vi "Auto Kettle Final.vi"() -> ()   [LabVIEW 2023]
uses:
  <vilib>/MakerHub/LINX/Public/Peripherals/Digital/Digital Read 1 Chan.vi
  <vilib>/MakerHub/LINX/Public/Peripherals/Digital/Digital Write 1 Chan.vi
  <vilib>/MakerHub/LINX/Public/Peripherals/Digital/Digital Read N Chans.vi
  <vilib>/MakerHub/LINX/Public/Peripherals/Digital/Digital Write N Chans.vi
  <vilib>/MakerHub/LINX/Private/Local IO/LinxDigitalRead.vi
  <vilib>/MakerHub/LINX/Public/Utilities/Check Channel.vi
  <vilib>/MakerHub/LINX/Private/Local IO/LinxDigitalWrite.vi
  <vilib>/MakerHub/LINX/Public/Utilities/Open Serial.vi
  <vilib>/MakerHub/LINX/Private/Utilties/Generate Error.vi
  <vilib>/MakerHub/LINX/LMH-LINX.lvlib
panel:
  out "Kettle OFF":bool
  in  "True":string
  in  "False":string
  out "Live LED":bool
  out "Error Out":errorcluster
  in  "Serial Port":refnum<visa-resource-name>="N/A"
  out "Measured Temperature":dbl
  out "Waveform Chart":dbl(graph)
  in  "stop":bool
  in  "Desired Temp":i32=40
  out "Kettle On":bool
  out "Kettle Temp":dbl(slide) scale=0.0..100.0
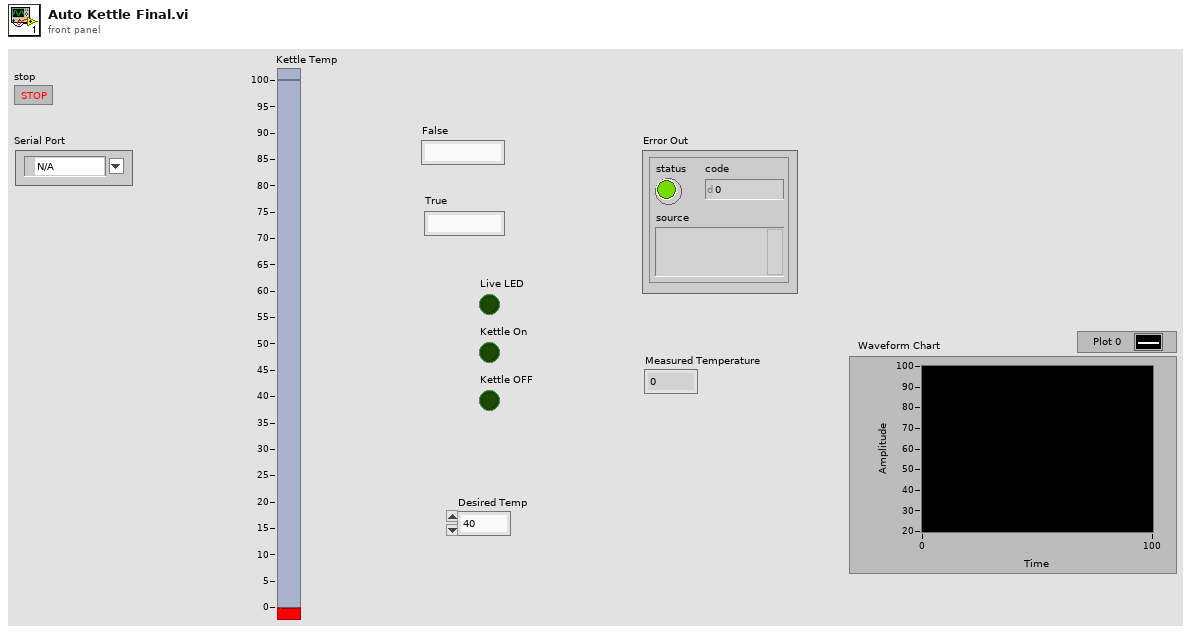
[diagram p1: front panel]
types:
  T1 = typedef "LMH-LINX.lvlib/LINX Ref.ctl" = cluster{"IO":T2, "Interface":T3, "LINX Device Config":T4}
  T2 = typedef "LMH-LINX.lvlib/Platform.ctl" = enum16{"Remote", "Local"}
  T3 = typedef "LMH-LINX.lvlib/Interface.ctl" = enum16{"Serial", "TCP"}
  T4 = typedef "LMH-LINX.lvlib/Device.lvlib/LINX Device Config.ctl" = cluster{"Interface":T3, "COM Port":refnum<visa-resource-name>, "TCP Configuration":T5, "Device Family":u8, "Device ID":u8, "Device Name":string, "TCP Ref":refnum<k5>, "Channels":T6}
  T5 = typedef "LMH-LINX.lvlib/Device.lvlib/TCP Config.ctl" = cluster{"IP Address":string, "Port":u16}
  T6 = typedef "LMH-LINX.lvlib/Channels.ctl" = cluster{"DI":u8[], "DO":u8[], "AI":u8[], "AO":u8[], "PWM":u8[], "QE":u8[], "UART":u8[], "I2C 2":u8[], "SPI":u8[], "CAN":u8[], "Servo":u8[], "AI Ref (V)":dbl, "AI Resolution (Bits)":u8, "AO Ref (V)":dbl, "AO Resolution (Bits)":u8}
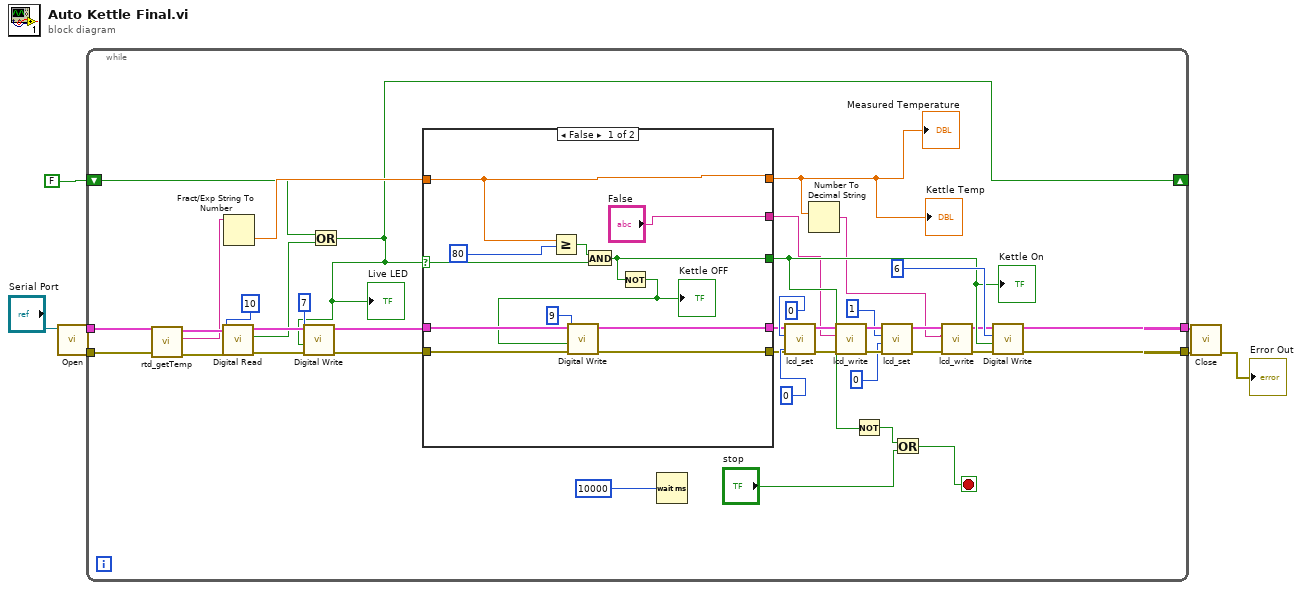
[diagram p0: block diagram]
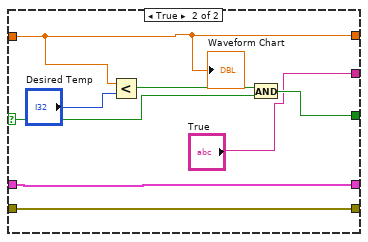
[diagram p2: hidden frame]
diagram:
  n1 = call-poly <vilib>:"Open.vi"("Serial Port"="Serial Port") -> ("Error Out"=w4:errorcluster, "LINX Resource"=w5:T1)  [unwired: 8 in, 1 out]
  n2 = while {
    shift-right: [w9] -> _
    shift-left: FALSE -> [w34]
    tunnel: w5 -> [w40]
    tunnel: w4 -> [w39]
    tunnel: [w20] -> w1
    tunnel: [w21] -> w2
    stop <- w45 stop-if-true
    n3 = call "rtd_getTemp.vi"("Error In"=w39, "LINX Resource"=w40) -> ("Error Out"=w38:errorcluster, "string"=w35:string, "LINX Resource 2"=w37:T1)  [unwired: 7 in]
    n4 = call-poly <vilib>:"Digital Read.vi"("Error In"=w38, "DI Channel"=10, "LINX Resource"=w37) -> ("Error Out"=w33:errorcluster, "DI Value"=w31:bool, "LINX Resource"=w32:T1)  [unwired: 6 in]
    n5 = Fract/Exp String To Number(string=w35) -> (number=w36:dbl)  [unwired: 3 in, 1 out]
    n6 = Or(x=w34, y=w31) -> (x .or. y?=w9:bool)
    "Live LED" <- w9
    n7 = call-poly <vilib>:"Digital Write.vi"("Error In"=w33, "Output Value"=w9, "DO Channel"=u8 7, "LINX Resource"=w32) -> ("Error Out"=w24:errorcluster, "LINX Resource"=w25:T1)  [unwired: 6 in]
    n8 = case shown="False" w9 {
      selector: w9 -> [w51 w62]
      tunnel: w36 -> [w57 w61]
      tunnel: [w57 w61] -> w8
      tunnel: [w49 w65] -> w41
      tunnel: w25 -> [w53 w63]
      tunnel: [w55 w63] -> w23
      tunnel: w24 -> [w52 w64]
      tunnel: [w54 w64] -> w22
      tunnel: ["False" "True"] -> w13
      frame False {
        n9 = Greater Or Equal?(x=w57, y=80 ("Numeric")) -> (x >= y?=w58:bool)
        n10 = And(x=w58, y=w51) -> (x .and. y?=w49:bool)
        n11 = Not(x=w49) -> (.not. x?=w48:bool)
        "Kettle OFF" <- w48
        n12 = call-poly <vilib>:"Digital Write.vi"("Error In"=w52, "Output Value"=w48, "DO Channel"=u8 9, "LINX Resource"=w53) -> ("Error Out"=w54:errorcluster, "LINX Resource"=w55:T1)  [unwired: 6 in]
      }
      frame True {
        n13 = Less?(x=w61, y="Desired Temp") -> (x < y?=w66:bool)
        n14 = And(x=w66, y=w62) -> (x .and. y?=w65:bool)
        "Waveform Chart" <- w61
      }
    }
    "Kettle Temp" <- w8
    "Kettle On" <- w41
    "Measured Temperature" <- w8
    n15 = Wait (ms)(milliseconds to wait=10000) -> ()  [unwired: 1 out]
    n16 = call "lcd_set.vi"("Error In"=w22, "Column"=0, "Row"=0, "LINX Resource"=w23) -> ("Error Out"=w27:errorcluster, "LINX Resource out"=w26:T1)  [unwired: 6 in]
    n17 = Number To Decimal String(number=w8) -> (decimal integer string=w12:string)  [unwired: 1 in]
    n18 = call "lcd_write.vi"("Error In"=w27, "string"=w13, "LINX Resource"=w26) -> ("Error Out"=w18:errorcluster, "LINX Resource out"=w19:T1)  [unwired: 7 in]
    n19 = Not(x=w41) -> (.not. x?=w46:bool)
    n20 = call "lcd_set.vi"("Error In"=w18, "Column"=0, "Row"=1, "LINX Resource"=w19) -> ("Error Out"=w17:errorcluster, "LINX Resource out"=w16:T1)  [unwired: 6 in]
    n21 = Or(x=w46, y="stop") -> (x .or. y?=w45:bool)
    n22 = call "lcd_write.vi"("Error In"=w17, "string"=w12, "LINX Resource"=w16) -> ("Error Out"=w15:errorcluster, "LINX Resource out"=w14:T1)  [unwired: 7 in]
    n23 = call-poly <vilib>:"Digital Write.vi"("Error In"=w15, "Output Value"=w41, "DO Channel"=6, "LINX Resource"=w14) -> ("Error Out"=w20:errorcluster, "LINX Resource"=w21:T1)  [unwired: 6 in]
  }
  n24 = call <vilib>:"Close.vi"("Error In"=w1, "LINX Resource"=w2) -> ("Error Out"=→"Error Out":errorcluster)  [unwired: 9 in]
